vi "ChargeDir.vi"(8 "AttackMap DVR In":T2, 10 "Origin":T1, 11 "Position":T1) -> (0 "AttackMap DVR Out":T2, 2 "Origin Out":T1, 3 "Direction Of Charge":T3)   [LabVIEW 2017, in "Atom.lvclass"]
uses:
  Atom.lvclass
  Type Defs/Direction Enum.ctl
  Type Defs/SB Type Defs.lvlib
  Common/Position.ctl
  Common/Common.lvlib
  AttackMap DVR.ctl
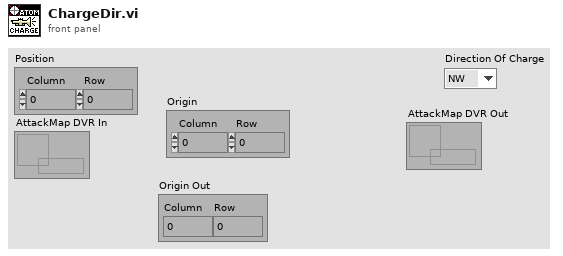
[diagram p1: front panel]
types:
  T1 = typedef "Common.lvlib/Position.ctl" = cluster{"Column":i32, "Row":i32}
  T2 = typedef "Atom.lvclass/AttackMap DVR.ctl" = refnum<data-value>
  T3 = typedef "SB Type Defs.lvlib/Direction Enum.ctl" = enum16{"NW", "N", "NE", "E", "SE", "S", "SW", "W"}
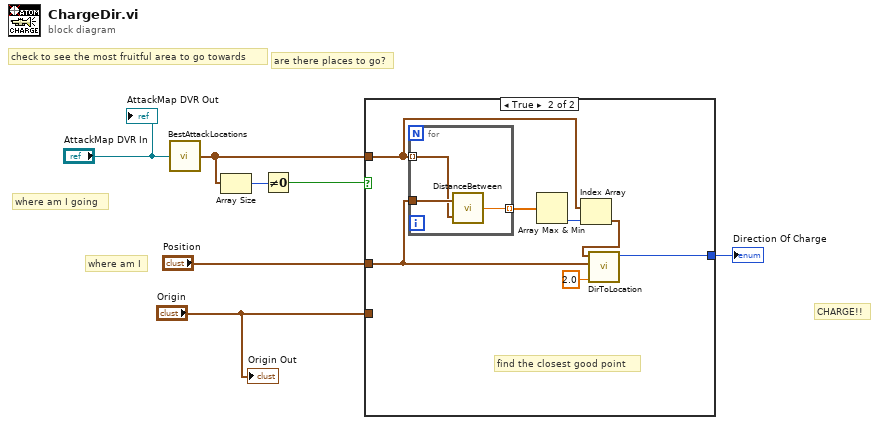
[diagram p0: block diagram]
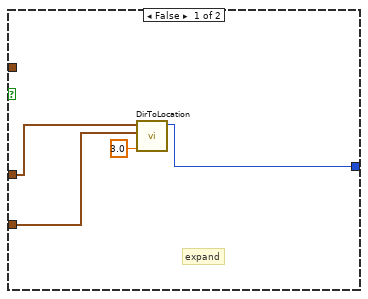
[diagram p2: hidden frame]
diagram:
  # "are there places to go?"
  # "CHARGE!!"
  # "where am I going"
  # "where am I"
  # "check to see the most fruitful area to go towards"
  n1 = call "BestAttackLocations.vi"("AttackMap DVR"="AttackMap DVR In") -> ("Locations"=w5:T1[])
  n2 = Array Size(array=w5) -> (size(s)=w4:i32)
  n3 = Not Equal To 0?(x=w4) -> (x != 0?=w3:bool)
  n4 = case shown="True" w3 {
    tunnel: [w8 w13] -> w7
    tunnel: "Position" -> [w10 w17]
    tunnel: w5 -> [_ w15]
    tunnel: "Origin" -> [w11 _]
    frame False {
      # "expand"
      n5 = call "DirToLocation.vi"("noise"=3.0, "Origin"=w11, "Position"=w10) -> ("Direction"=w8:T3)  [unwired: 8 in]
    }
    frame True {
      # "find the closest good point"
      n6 = for {
        tunnel: w15 -> [w20] mode=indexing
        tunnel: w17 -> [w21]
        tunnel: [w19] -> w16 mode=indexing
        n7 = call "DistanceBetween.vi"("B"=w20, "A"=w21) -> ("Dist(A,B)"=w19:dbl)
      }
      n8 = Array Max & Min(array=w16) -> (min index (indices)=w18:i32)  [unwired: 3 out]
      n9 = Index Array(array=w15, index=w18) -> (element=w14:T1)
      n10 = call "DirToLocation.vi"("noise"=2.0, "Origin"=w17, "Position"=w14) -> ("Direction"=w13:T3)  [unwired: 8 in]
    }
  }
  "Direction Of Charge" <- w7
  "Origin Out" <- "Origin"
  "AttackMap DVR Out" <- "AttackMap DVR In"
